vi "MasterSlavePatternVoorbeeld.vi"() -> ()   [LabVIEW 2019]
doc: "Use this template to build a master/slave design pattern. The master loop always executes. It notifies one or more slave loops to execute their code. The slave loop(s) continue executing until they complete, then wait for another notification. Contrast this with the Producer/Consumer pattern in which the consumer loops execute only when they have data in their queue."
panel:
  in  "Master Loop Notification Message":string="instruction"
  out "Slave Loop Notification Message":string
  in  "Sent to Slave Loop":bool
  in  "stop":bool
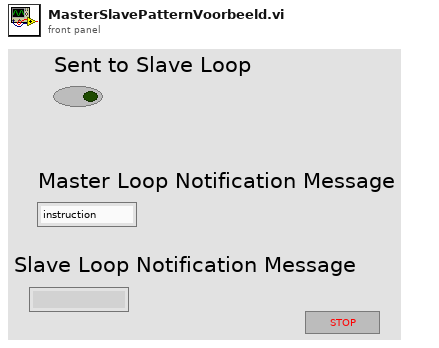
[diagram p1: front panel]
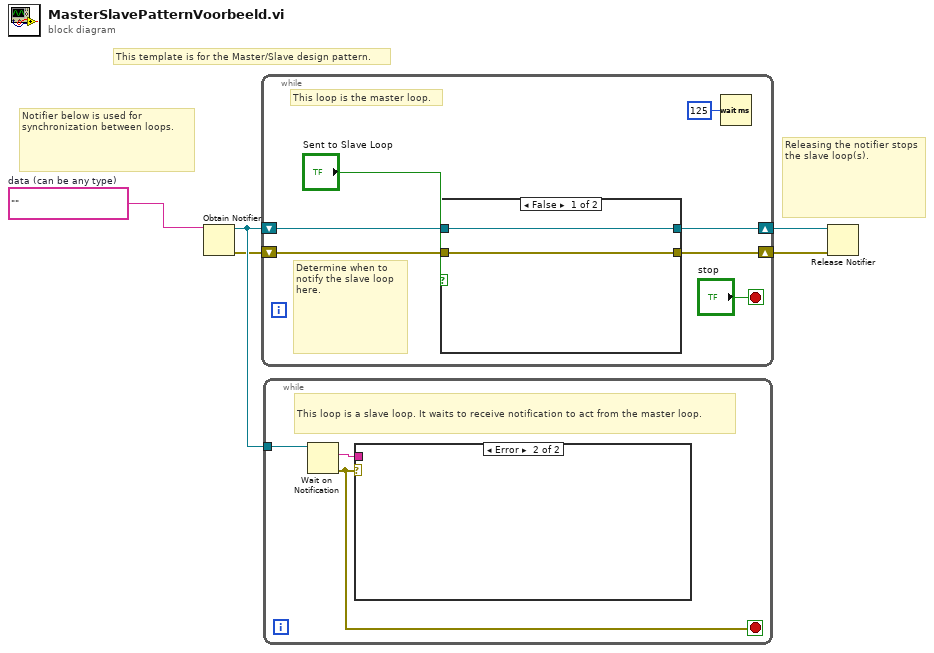
[diagram p0: block diagram]
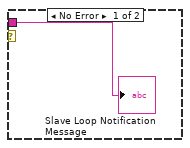
[diagram p2: hidden frame]
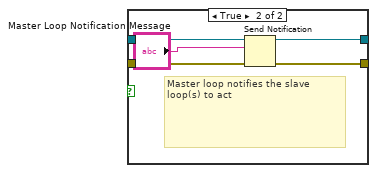
[diagram p3: hidden frame]
diagram:
  w1 = ""  # data (can be any type)
  # "Releasing the notifier stops the slave loop(s)."
  # "This template is for the Master/Slave design pattern."
  # "Notifier below is used for  synchronization between loops."
  n1 = Obtain Notifier(notification data type=w1) -> (notifier out=w5:refnum<notifier>, error out=w4:errorcluster)  [unwired: 2 in, 2 out]
  n2 = while {
    shift-right: [w10] -> w3
    shift-left: w4 -> [w9]
    shift-right: [w8] -> w2
    shift-left: w5 -> [w11]
    stop <- "stop" stop-if-true
    # "Determine when to notify the slave loop here."
    # "This loop is the master loop."
    n3 = case shown="False" "Sent to Slave Loop" {
      tunnel: w11 -> [w13 w19]
      tunnel: [w14 w18] -> w10
      tunnel: w9 -> [w14 w17]
      tunnel: [w13 w16] -> w8
      frame False {
      }
      frame True {
        # "Master loop notifies the slave loop(s) to act"
        n4 = Send Notification(notification="Master Loop Notification Message", notifier=w19, error in (no error)=w17) -> (notifier out=w16:refnum<notifier>, error out=w18:errorcluster)
      }
    }
    n5 = Wait (ms)(milliseconds to wait=u32 125) -> ()  [unwired: 1 out]
  }
  n6 = while {
    tunnel: w5 -> [w22]
    stop <- w21 stop-if-true
    # "This loop is a slave loop. It waits to receive notification to act from the master loop."
    n7 = Wait on Notification(notifier=w22) -> (notification=w20:string, error out=w21:errorcluster)  [unwired: 1 in, 4 out]
    n8 = case shown="Error" w21 {
      tunnel: w20 -> [w23 _]
      frame No Error {
        "Slave Loop Notification Message" <- w23
      }
      frame Error {
      }
    }
  }
  n9 = Release Notifier(notifier=w2, error in (no error)=w3) -> ()  [unwired: 4 out]
